vi "Connect_to_BSA_IP.vi"(3 "Force Reconnect":bool) -> (0 "error out":errorcluster, 1 "BSA":refnum<k7>)   [LabVIEW 2016]
uses:
  Globals/LDA_meas_global_1.vi
panel:
  out "First error":errorcluster
  in  "BSACtrl.IBSA":refnum<k7>
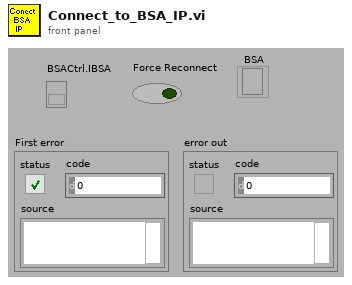
[diagram p1: front panel]
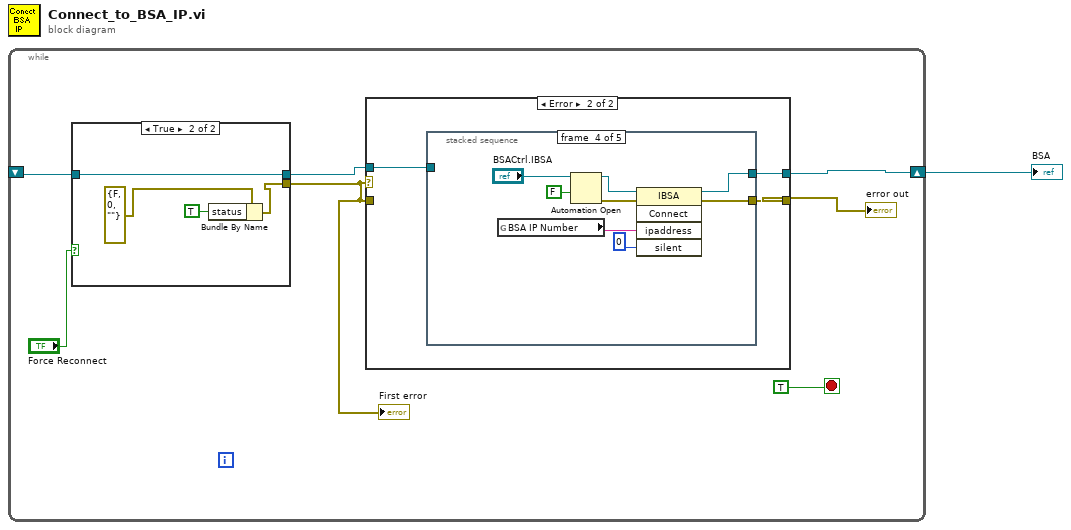
[diagram p0: block diagram]
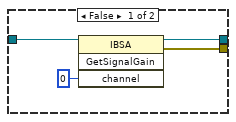
[diagram p2: hidden frame]
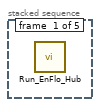
[diagram p4: hidden frame]
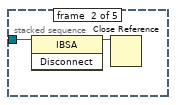
[diagram p5: hidden frame]
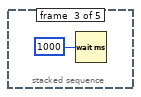
[diagram p6: hidden frame]
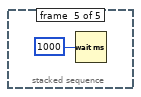
[diagram p7: hidden frame]
diagram:
  n1 = while {
    shift-right: [w5] -> w1
    shift-left: _ -> [w6]
    stop <- TRUE stop-if-true
    n2 = case shown="True" "Force Reconnect" {
      tunnel: [w11 w14] -> w8
      tunnel: [w10 w16] -> w7
      tunnel: w6 -> [w9 w16]
      frame False {
        n3 = invoke class="IBSA" method="GetSignalGain"(reference=w9, "channel"=0) -> (reference out=w10:refnum<k7>, error out=w11:errorcluster)  [unwired: 2 in, 2 out]
      }
      frame True {
        n4 = Bundle By Name(cluster=errorcluster {"status"=FALSE, "code"=0, "source"=""} ("error out"), "status"=TRUE) -> (w14:errorcluster)
      }
    }
    "First error" <- w8
    n5 = case shown="Error" w8 {
      tunnel: [w18 w21] -> w5
      tunnel: w7 -> [w18 w19]
      tunnel: [w17 w20] -> w4
      tunnel: w8 -> [w17 _]
      frame No Error {
      }
      frame Error {
        n6 = stacked-sequence {
          tunnel: w19 -> [_ w23 _ _ _]
          tunnel: [_ _ _ w26 _] -> w21
          tunnel: [_ _ _ w25 _] -> w20
          frame #0 {
            n7 = call "Run_EnFlo_Hub.vi"() -> ()  [unwired: 1 in, 7 out]
          }
          frame #1 {
            n8 = invoke class="IBSA" method="Disconnect"(reference=w23) -> (reference out=w22:refnum<k7>)  [unwired: 2 in, 2 out]
            n9 = Close Reference(reference=w22) -> ()  [unwired: 1 in, 1 out]
          }
          frame #2 {
            n10 = Wait (ms)(milliseconds to wait=u32 1000) -> ()  [unwired: 1 out]
          }
          frame #3 {
            n11 = global read "LDA_meas_global_1.vi" "BSA IP Number"() -> (w28:string)
            n12 = Automation Open(Automation Refnum="BSACtrl.IBSA", 9:FALSE ("open new instance (false)")) -> (Automation Refnum=w31:refnum<k7>, error out=w30:errorcluster)  [unwired: 2 in]
            n13 = invoke class="IBSA" method="Connect"(reference=w31, error in=w30, "ipaddress"=w28, "silent"=0) -> (reference out=w26:refnum<k7>, error out=w25:errorcluster)  [unwired: 1 in, 3 out]
          }
          frame #4 {
            n14 = Wait (ms)(milliseconds to wait=u32 1000) -> ()  [unwired: 1 out]
          }
        }
      }
    }
    "error out" <- w4
  }
  "BSA" <- w1
